vi "Util_MetersToRounds.vi"(2 "distance (m) robot":dbl) -> (0 "rotations gear":dbl)   [LabVIEW 2009, in "OWNCAN.lvlib"]
doc: "Converts distance traveled by the robot into number of rotations of the output shaft."
uses:
  OWNCAN.lvlib
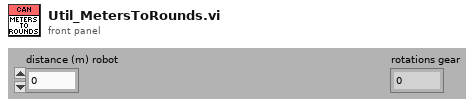
[diagram p1: front panel]
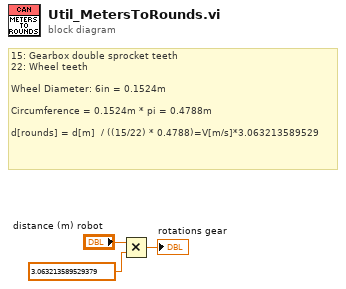
[diagram p0: block diagram]
diagram:
  # "15: Gearbox double sprocket teeth\n22: Wheel teeth\n\nWheel Diameter: 6in = 0.1524m\n\nCircumference = 0.1524m * pi = 0.4788m\n\nd[rounds] = d[m]  / ((15/22) * 0.4788)=V[m/s]*3.063213589529"
  n1 = Multiply(x="distance (m) robot", y=3.063213589529379) -> (x*y=→"rotations gear":dbl)
